vi "Up_Calib_DrawCycle.vi"(10 "CirclesDataIn":T1, 11 "ImageIn":T2) -> (3 "Image Out":T2)   [LabVIEW 2019]
uses:
  <vilib>/vision/Image Controls.llb/IMAQ Image.ctl
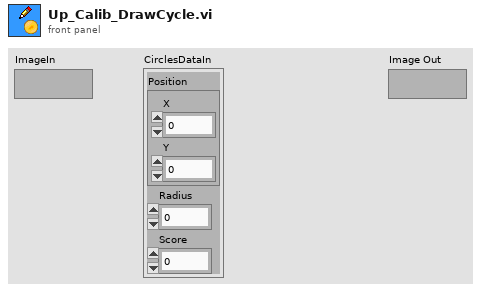
[diagram p1: front panel]
types:
  T1 = cluster{"Position":cluster{"X":sgl, "Y":sgl}, "Radius":dbl, "Score":dbl}
  T2 = typedef "IMAQ Image.ctl" = refnum<image>
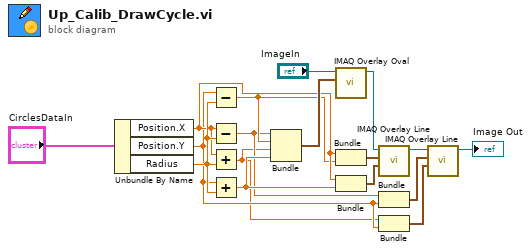
[diagram p0: block diagram]
diagram:
  n1 = Unbundle By Name("CirclesDataIn") -> ("Position.X"=w15:sgl, "Position.Y"=w10:sgl, "Radius"=w17:dbl)
  n2 = Subtract(x=w10, y=w17) -> (x-y=w13:dbl)
  n3 = Subtract(x=w15, y=w17) -> (x-y=w9:dbl)
  n4 = Add(x=w15, y=w17) -> (x+y=w8:dbl)
  n5 = Add(x=w10, y=w17) -> (x+y=w12:dbl)
  n6 = Bundle(w9, w13, w8, w12) -> (w16:cluster{dbl, dbl, dbl, dbl})  [unwired: 1 in]
  n7 = call "IMAQ Overlay Oval"("Bounding Rectangle"=w16, "Image"="ImageIn") -> ("Image Out"=w5:T2)  [unwired: 8 in, 1 out]
  n8 = Bundle("X"=w15, w13) -> (w14:cluster{"X":sgl, dbl})  [unwired: 1 in]
  n9 = Bundle("X"=w15, w12) -> (w11:cluster{"X":sgl, dbl})  [unwired: 1 in]
  n10 = call "IMAQ Overlay Line"("End Point"=w11, "Start Point"=w14, "Image"=w5) -> ("Image Out"=w4:T2)  [unwired: 7 in, 1 out]
  n11 = Bundle(w9, "Y"=w10) -> (w7:cluster{dbl, "Y":sgl})  [unwired: 1 in]
  n12 = Bundle(w8, "Y"=w10) -> (w6:cluster{dbl, "Y":sgl})  [unwired: 1 in]
  n13 = call "IMAQ Overlay Line"("End Point"=w6, "Start Point"=w7, "Image"=w4) -> ("Image Out"=→"Image Out":T2)  [unwired: 7 in, 1 out]
